vi "8_VI_Longitude_convert.vi"(10 "Longitude (dddmm.mmmmm)":string) -> (1 "Longitude":dbl)   [LabVIEW 2019]
doc: "SubVI der omdanner NMEA string til Longitude værdi\n\nBygget på VI diagram fra dokumentet: \nZED-F9P RTK GPS E2019\nMechatronic challenge group 10\nAarhus University\nThe 21st May 2019"
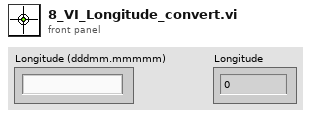
[diagram p1: front panel]
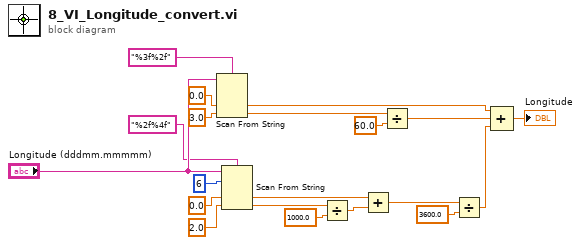
[diagram p0: block diagram]
diagram:
  n1 = Scan From String(format string="%3f%2f", input string="Longitude (dddmm.mmmmm)", default 1=0.0 ("default value 1"), default 2=3.0 ("default value 2")) -> (output 1=w10:dbl, output 2=w9:dbl)  [unwired: 2 in, 3 out]
  n2 = Scan From String(format string="%2f%4f", input string="Longitude (dddmm.mmmmm)", initial scan location=u32 6, default 1=0.0 ("default value 1"), default 2=2.0 ("default value 2")) -> (output 1=w7:dbl, output 2=w6:dbl)  [unwired: 1 in, 3 out]
  n3 = Divide(x=w6, y=1000.0) -> (x/y=w14:dbl)
  n4 = Add(x=w7, y=w14) -> (x+y=w13:dbl)
  n5 = Divide(x=w9, y=60.0) -> (x/y=w12:dbl)
  n6 = Divide(x=w13, y=3600.0) -> (x/y=w11:dbl)
  n7 = Compound Arithmetic op=ADD(w10, w12, w11) -> (→"Longitude":dbl)
